vi "onDeserializeParameters.vi"(8 "error in (no error)":errorcluster, 10 "Variant":variant, 11 "RequirementMap in":refnum<class "RequirementMap.lvclass">) -> (0 "error out":errorcluster, 3 "RequirementMap out":refnum<class "RequirementMap.lvclass">)   [LabVIEW 2021, in "Bananas.lvlib" / "RequirementMap.lvclass"]
uses:
  RequirementMap.lvclass
  RequirementMap.lvclass/RequirementMap.ctl
  <vilib>/LabVIEW Open Source Project/Data Manipulation/TypeDescriptor/TypeDescriptor_GetType.vi
  <vilib>/LabVIEW Open Source Project/Data Manipulation/TypeDescriptor/TypeDescriptor_GetName.vi
  <vilib>/LabVIEW Open Source Project/Data Manipulation/TypeDescriptor/TypeDescriptor_GetPString.vi
  <vilib>/Utility/GetType.llb/Get Type Code from I16 Array And Pos.vi
  BananaPeel/BananaPeel.lvclass
  <vilib>/LabVIEW Open Source Project/Data Manipulation/Variant/OpenVariant.lvlib
  <vilib>/LabVIEW Open Source Project/OpenURI/uri/URI.lvclass
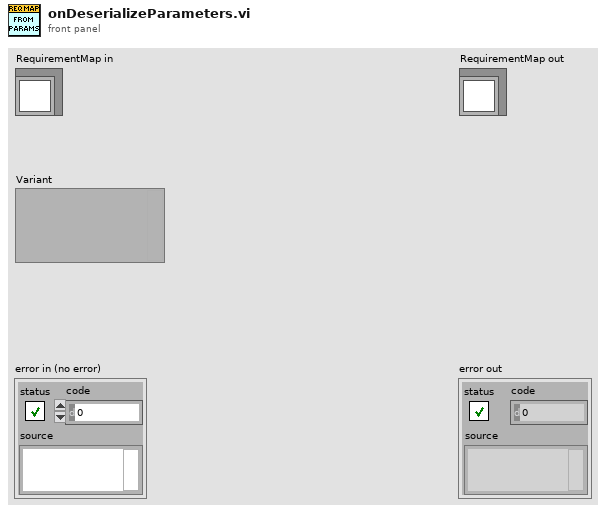
[diagram p1: front panel]
types:
  T1 = typedef "Type Enum.ctl" = enum8{"Void", "I8", "I16", "I32", "I64", "U8", "U16", "U32", "U64", "Single Float", "Double Float", "Extended Float", "Single Complex", "Double Complex", "Extended Complex", "Enum I8 NEVER", "Enum I16 NEVER", "Enum I32 NEVER", "Enum I64 NEVER", "Enum U8", "Enum U16", "Enum U32", "Enum U64", "Single Float With Unit", "Double Float With Unit", "Extended Float With Unit", "Single Complex With Unit", "Double Complex With Unit", "Extended Complex With Unit", "boolU16", "Boolean", "String", "Handle", "Path", "Picture", "C String", "Pascal String", "Tag", "SubString", "Array", "SubArray", "Cluster", "Numeric Cluster", "Variant", "LV Variant", "Measure Data (waveform)", "Refnum", "ExtData", "function", "Typedef", "Poly VI", "bad wire", "LabVIEW Class Instance"}
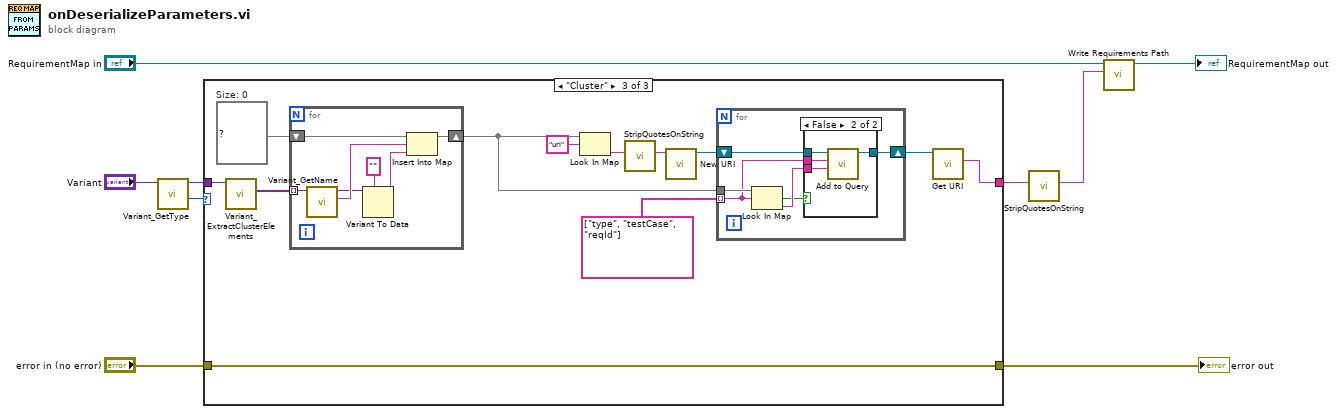
[diagram p0: block diagram]
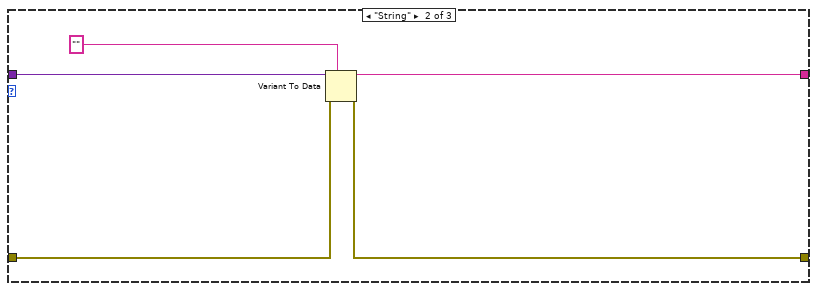
[diagram p3: hidden frame]
diagram:
  n1 = call <vilib>:"Variant_GetType.vi"("Variant"="Variant") -> ("Type Enum"=w3:T1, "Variant dup"=w1:variant)  [unwired: 8 in, 1 out]
  n2 = case shown="\"Cluster\"" w3 {
    tunnel: [_ w15 w25] -> w6
    tunnel: "error in (no error)" -> [w10 w14 w24]
    tunnel: [w10 w13 w24] -> w4
    tunnel: w1 -> [_ w11 w23]
    frame Default {
    }
    frame "String" {
      n3 = Variant To Data(error in=w14, type="", Variant=w11) -> (data=w15:string, error out=w13:errorcluster)
    }
    frame "Cluster" {
      w21 = map{string, string} {}  # Size: 0
      n4 = call <vilib>:"Variant_ExtractClusterElements.vi"("Cluster"=w23) -> ("Elements"=w22:variant[])  [unwired: 8 in, 2 out]
      n5 = for {
        tunnel: w22 -> [w45] mode=indexing
        shift-right: [w43] -> w18
        shift-left: w21 -> [w42]
        n6 = call <vilib>:"Variant_GetName.vi"("Variant"=w45) -> ("Name"=w44:string, "Variant dup"=w40:variant)  [unwired: 8 in, 1 out]
        n7 = Variant To Data(type="" ("name"), Variant=w40) -> (data=w39:string)  [unwired: 1 in, 1 out]
        n8 = Insert Into Map(map in=w42, key=w44, value=w39) -> (map out=w43:map{string, string})  [unwired: 2 out]
      }
      n9 = Look In Map(map=w18, key="uri" ("name")) -> (value=w19:string)  [unwired: 1 in, 1 out]
      n10 = call "StripQuotesOnString.vi"("String"=w19) -> ("Unquoted String"=w27:string)  [unwired: 10 in]
      n11 = call <vilib>:"New URI.vi"("URI"=w27) -> ("URI"=w26:refnum<class "URI.lvclass">)  [unwired: 9 in, 1 out]
      n12 = for {
        tunnel: w18 -> [w32]
        tunnel: string[] ["type", "testCase", "reqId"] -> [w29] mode=indexing
        shift-right: [w28] -> w17
        shift-left: w26 -> [w33]
        n13 = Look In Map(map=w32, key=w29) -> (key not found?=w30:bool, value=w31:string)  [unwired: 1 in]
        n14 = case shown="False" w30 {
          tunnel: w33 -> [w34 w38]
          tunnel: [w34 w37] -> w28
          tunnel: w29 -> [_ w36]
          tunnel: w31 -> [_ w35]
          frame True {
          }
          frame False {
            n15 = call <vilib>:"Add to Query.vi"("value"=w35, "key"=w36, "URI in"=w38) -> ("URI out"=w37:refnum<class "URI.lvclass">)  [unwired: 7 in, 1 out]
          }
        }
      }
      n16 = call <vilib>:"Get URI.vi"("URI in"=w17) -> ("URI String"=w25:string)  [unwired: 8 in, 2 out]
    }
  }
  "error out" <- w4
  n17 = call "StripQuotesOnString.vi"("String"=w6) -> ("Unquoted String"=w9:string)  [unwired: 10 in]
  n18 = call "Write Requirements Path.vi"("URI"=w9, "Project in"="RequirementMap in") -> ("Project out"=→"RequirementMap out":refnum<class "RequirementMap.lvclass">)  [unwired: 9 in]
